vi "Post Submit.vi"(0 "CommitNIPKG_LV in":refnum<class "CommitNIPKG_LV.lvclass">) -> (4 "CommitNIPKG_LV out":refnum<class "CommitNIPKG_LV.lvclass">)   [LabVIEW 2017, in "CL_G3_VIComponentBuilder.lvlib" / "CommitNIPKG_LV.lvclass"]
doc: "All actions taken after comitting the export."
uses:
  CommitNIPKG_LV.lvclass
  C:/builds/Component BuilderBT/SrcDist/Commit Behavior/Commit/Commit.lvclass
  Commit/Commit.lvclass/Commit.ctl
  Commit/Accessors/Write Commit Operation Errors.vi
  Commit/Commit.lvclass
  <userlib>/_Cirrus Logic/NI Package Manager API/Source/TCS_NIPKG_API.lvlib
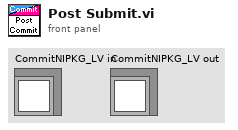
[diagram p1: front panel]
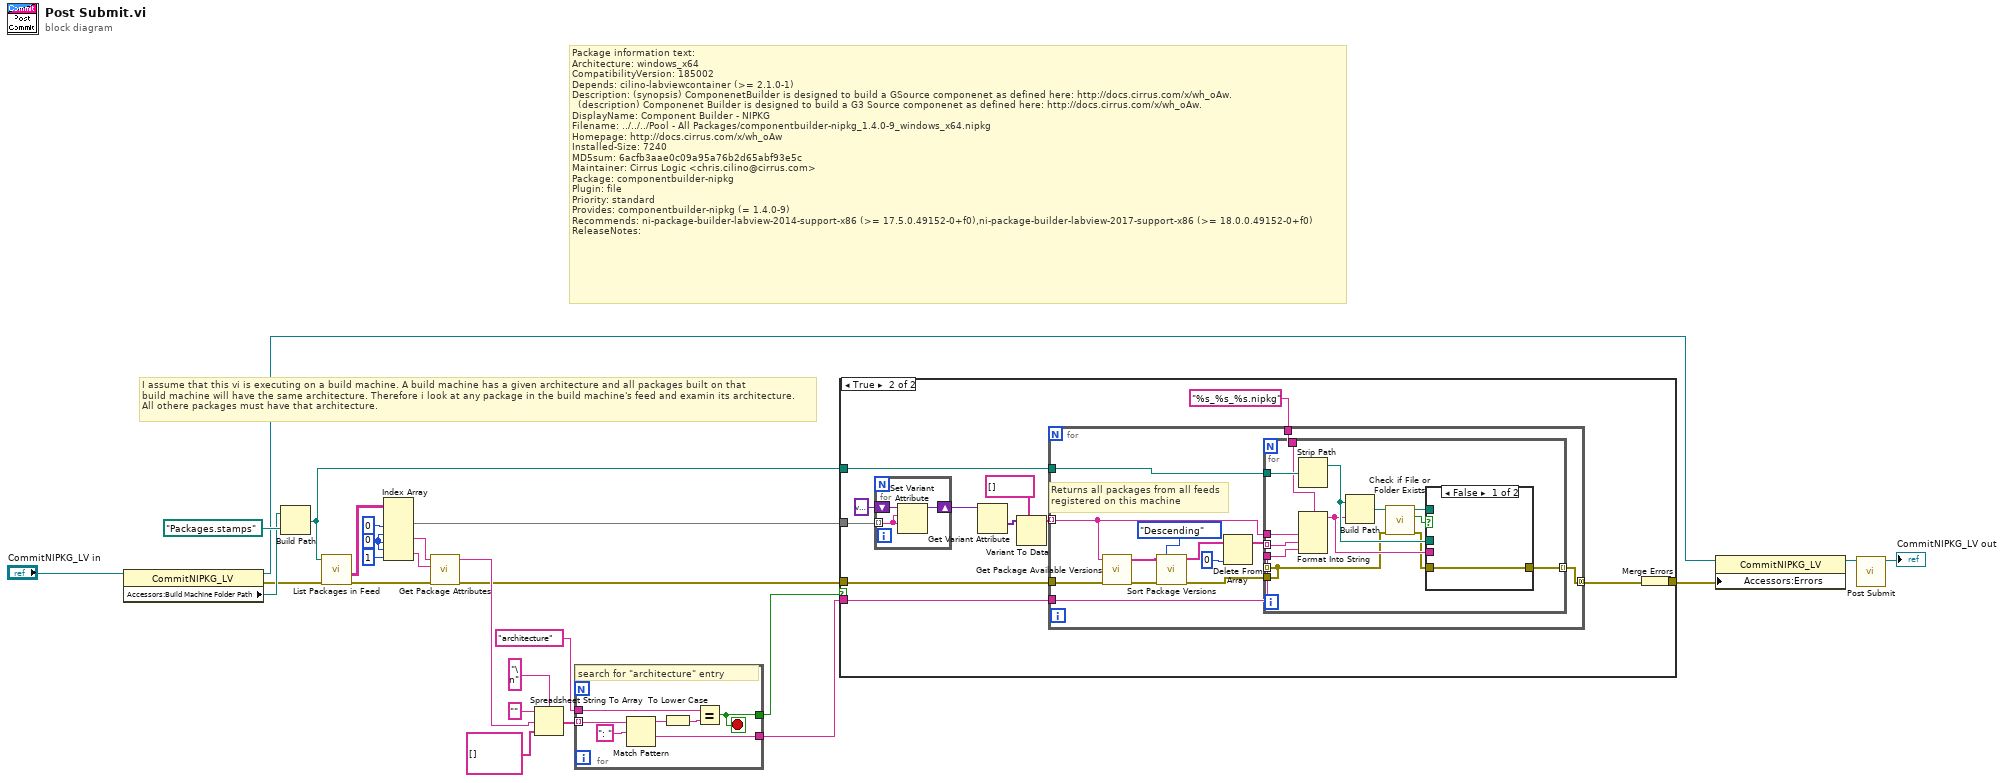
[diagram p0: block diagram]
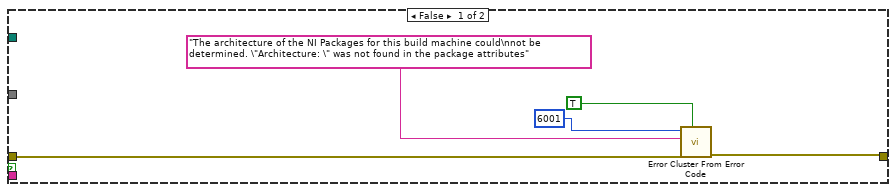
[diagram p2: hidden frame]
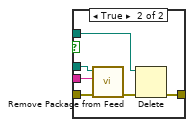
[diagram p3: hidden frame]
diagram:
  w8 = 0 ("index (row)")
  # "Package information text:\nArchitecture: windows_x64\nCompatibilityVersion: 185002\nDepends: cilino-labviewcontainer (>= 2.1.0-1)\nDescription: (synopsis) ComponenetBuilder is designed to build a GSource componenet as defined here: http://docs.cirrus.com/x/wh_oAw.\n  (description) Componenet Builder is designed to build a G3 Source componenet as defined here: http://docs.cirrus.com/x/wh_oAw.\nDisplayName: Component Builder - NIPKG\nFilename: ../../../Pool - All Packages/componentbuilder-nipkg_1.4.0-9_windows_x64.nipkg\nHomepage: http://docs.cirrus.com/x/wh_oAw\nInstalled-Size: 7240\nMD5sum: 6acfb3aae0c09a95a76b2d65abf93e5c\nMaintainer: Cirrus Logic <chris.cilino@cirrus.com>\nPackage: componentbuilder-nipkg\nPlugin: file\nPriority: standard\nProvides: componentbuilder-nipkg (= 1.4.0-9)\nRecommends: ni-package-builder-labview-2014-support-x86 (>= 17.5.0.49152-0+f0),ni-package-builder-labview-2017-support-x86 (>= 18.0.0.49152-0+f0)\nReleaseNotes:"
  # "I assume that this vi is executing on a build machine. A build machine has a given architecture and all packages built on that \nbuild machine will have the same architecture. Therefore i look at any package in the build machine's feed and examin its architecture.\nAll othere packages must have that architecture."
  n1 = property class="CommitNIPKG_LV"(reference="CommitNIPKG_LV in") -> (reference out=w21:refnum<class "CommitNIPKG_LV.lvclass">, error out=w19:errorcluster, "Accessors:Build Machine Folder Path"=w20:path)  [unwired: 1 in]
  n2 = Build Path(base path=w20, name or relative path=path "Packages.stamps" ("feed stamp filepath")) -> (appended path=w24:path)
  n3 = call <userlib>:"List Packages in Feed.vi"("error in"=w19, "feed stamp filepath"=w24) -> ("error out"=w22:errorcluster, "package table"=w18:string[][])  [unwired: 7 in, 1 out]
  n4 = Index Array(array=w18, index (col) #1=0 ("disabled index (col)"), index (row) #2=w8, index (col) #2=w8, index (row) #3=w8, index (col) #3=1 ("index (row)")) -> (element #1=w16:string[], element #2=w6:string, element #3=w5:string)  [unwired: 1 in]
  n5 = call <userlib>:"Get Package Attributes.vi"("error in"=w22, "version"=w5, "package name"=w6) -> ("error out"=w11:errorcluster, "Package Attributes (specific version)"=w12:string)  [unwired: 5 in, 2 out]
  n6 = Spreadsheet String To Array(delimiter (Tab)="\n", format string="", spreadsheet string=w12, array type (2D Dbl)=string[] []) -> (array=w4:string[])
  n7 = for {
    tunnel: w4 -> [w32] mode=indexing
    tunnel: [w29] -> w3
    tunnel: "architecture" ("x") -> [w28]
    tunnel: [w27] -> w1
    stop <- w27 stop-if-true
    # "search for \"architecture\" entry"
    n8 = Match Pattern(string=w32, regular expression=": ") -> (before substring=w31:string, after substring=w29:string)  [unwired: 1 in, 2 out]
    n9 = To Lower Case(string=w31) -> (all lower case string=w30:string)
    n10 = Equal?(x=w28, y=w30) -> (x = y?=w27:bool)
  }
  n11 = case shown="True" w1 {
    tunnel: w24 -> [_ w50]
    tunnel: w16 -> [_ w49]
    tunnel: w11 -> [w34 w43]
    tunnel: [w35 w41] -> w9
    tunnel: w3 -> [_ w40]
    frame False {
      n12 = call <vilib>:"Error Cluster From Error Code.vi"("show call chain? (False)"=TRUE, "error in (no error)"=w34, "error message (\"\")"="The architecture of the NI Packages for this build machine could\nnot be determined. \"Architecture: \" was not found in the package attributes" ("error message (\"\")"), "error code (0)"=6001) -> ("error out"=w35:errorcluster)  [unwired: 5 in]
    }
    frame True {
      n13 = for {
        tunnel: w49 -> [w51] mode=indexing
        shift-right: [w53] -> w47
        shift-left: variant ("Variant") -> [w52]
        n14 = Set Variant Attribute(Variant=w52, name=w51, value=w51) -> (Variant out=w53:variant)  [unwired: 1 in, 2 out]
      }
      n15 = Get Variant Attribute(Variant=w47) -> (values=w46:variant[])  [unwired: 3 in, 3 out]
      n16 = Variant To Data(type=string[] [], Variant=w46) -> (data=w44:string[])  [unwired: 1 in, 1 out]
      n17 = for {
        tunnel: w44 -> [w63] mode=indexing
        tunnel: w50 -> [w64]
        tunnel: w40 -> [w62]
        tunnel: w43 -> [w61]
        tunnel: [w60] -> w42 mode=concatenating
        tunnel: "%s_%s_%s.nipkg" ("format string") -> [w59]
        # "Returns all packages from all feeds \nregistered on this machine"
        n18 = call <userlib>:"Get Package Available Versions.vi"("error in"=w61, "package name"=w63) -> ("error out"=w55:errorcluster, "Versions"=w58:string[])  [unwired: 8 in]
        n19 = call <userlib>:"Sort Package Versions.vi"("Package Versions"=w58, "Sort Order"=enum16{"Ascending", "Descending"}."Descending", "error in"=w55) -> ("Sorted Versions"=w56:string[], "error out"=w54:errorcluster)  [unwired: 9 in, 2 out]
        n20 = Delete From Array(array=w56, index=0) -> (array with subset deleted=w65:string[])  [unwired: 1 in, 1 out]
        n21 = for {
          tunnel: w65 -> [w75] mode=indexing
          tunnel: w64 -> [w79]
          tunnel: w63 -> [w76]
          tunnel: [w77] -> w60 mode=indexing
          tunnel: w62 -> [w74]
          tunnel: [w67] -> _ mode=indexing
          tunnel: w59 -> [w72]
          tunnel: w54 -> [w67]
          n22 = Strip Path(path=w79) -> (stripped path=w78:path)  [unwired: 1 out]
          n23 = Format Into String(format string=w72, w76, w75, w74) -> (resulting string=w73:string)  [unwired: 2 in, 1 out]
          n24 = Build Path(base path=w78, name or relative path=w73) -> (appended path=w71:path)
          n25 = call <vilib>:"Check if File or Folder Exists.vi"("error in (no error)"=w67, "path"=w71) -> ("error out"=w68:errorcluster, "file or folder exists?"=w69:bool, "dup path"=w70:path)  [unwired: 7 in]
          n26 = case shown="False" w69 {
            tunnel: w78 -> [_ w86]
            tunnel: [w80 w84] -> w77
            tunnel: w73 -> [_ w83]
            tunnel: w68 -> [w80 w82]
            tunnel: w70 -> [_ w81]
            frame False {
            }
            frame True {
              n27 = call <userlib>:"Remove Package from Feed.vi"("error in"=w82, "package filename"=w83, "feed folderpath"=w86) -> ("error out"=w85:errorcluster)  [unwired: 8 in]
              n28 = Delete(path (use dialog)=w81, error in=w85) -> (error out=w84:errorcluster)  [unwired: 3 in, 2 out]
            }
          }
        }
      }
      n29 = Merge Errors(w42) -> (w41:errorcluster)
    }
  }
  n30 = property class="CommitNIPKG_LV"(reference=w21, "Accessors:Errors"=w9) -> (reference out=w10:refnum<class "CommitNIPKG_LV.lvclass">)  [unwired: 1 in, 1 out]
  n31 = call-parent "Post Submit.vi"("Commit in"=w10) -> ("Commit out"=→"CommitNIPKG_LV out":refnum<class "CommitNIPKG_LV.lvclass">)  [unwired: 14 in]
